vi "Update Class Properties.vi"(8 "error in (no error)":errorcluster, 11 "QControl Creation in":refnum<class "QControl Creation.lvclass">) -> (0 "error out":errorcluster, 3 "QControl Creation (dup)":refnum<class "QControl Creation.lvclass">)   [LabVIEW 2020, in "QControl Creation.lvclass"]
doc: "<b> </b> <b> </b>\n©2016 Q Software Innovations, LLC (QSI)\nwritten by Quentin Alldredge\nproduced in LabVIEW 2015\n\nsupport@qsoftwareinnovations.com\nwww.qsoftwareinnovations.com\n\nAll rights reserved.\n\nRedistribution and use in source and binary forms, with or without modification, are permitted provided that the following conditions are met:\n\n * Redistributions of source code must retain the above copyright notice, this list of conditions and the following disclaimer.\n * Redistributions in binary form must reproduce the above copyright notice, this list of conditions and the following disclaimer in the documentation and/or other materials provided with the distribution.\n * Neither the name of Q Software Innovations, LLC. nor the names of its contributors may be used to endorse or promote products derived from this software without specific prior written permission.\n\nTHIS SOFTWARE IS PROVIDED BY THE COPYRIGHT HOLDERS AND CONTRIBUTORS \"AS IS\" AND ANY EXPRESS OR IMPLIED WARRANTIES, INCLUDING, BUT NOT LIMITED TO, THE IMPLIED WARRANTIES OF MERCHANTABILITY AND FITNESS FOR A PARTICULAR PURPOSE ARE DISCLAIMED. IN NO EVENT SHALL THE COPYRIGHT OWNER OR CONTRIBUTORS BE LIABLE FOR ANY DIRECT, INDIRECT, INCIDENTAL, SPECIAL, EXEMPLARY, OR CONSEQUENTIAL DAMAGES (INCLUDING, BUT NOT LIMITED TO, PROCUREMENT OF SUBSTITUTE GOODS OR SERVICES; LOSS OF USE, DATA, OR PROFITS; OR BUSINESS INTERRUPTION) HOWEVER CAUSED AND ON ANY THEORY OF LIABILITY, WHETHER IN CONTRACT, STRICT LIABILITY, OR TORT (INCLUDING NEGLIGENCE OR OTHERWISE) ARISING IN ANY WAY OUT OF THE USE OF THIS SOFTWARE, EVEN IF ADVISED OF THE POSSIBILITY OF SUCH DAMAGE."
uses:
  QControl Creation.lvclass
  QControl Creation.lvclass/QControl Creation.ctl
  New QControl Info/New QControl Info.lvclass/New QControl Info.ctl
  New QControl Info/Read Localized Name.vi
  New QControl Info/Read Description.vi
  <vilib>/Utility/error.llb/Error Cluster From Error Code.vi
  <vilib>/ErrorRing/Error Ring.xnode
  New QControl Info/New QControl Info.lvclass
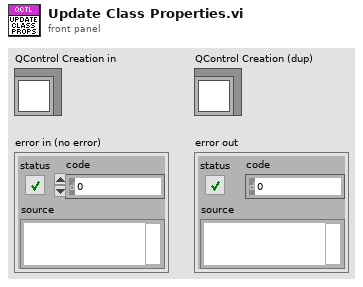
[diagram p1: front panel]
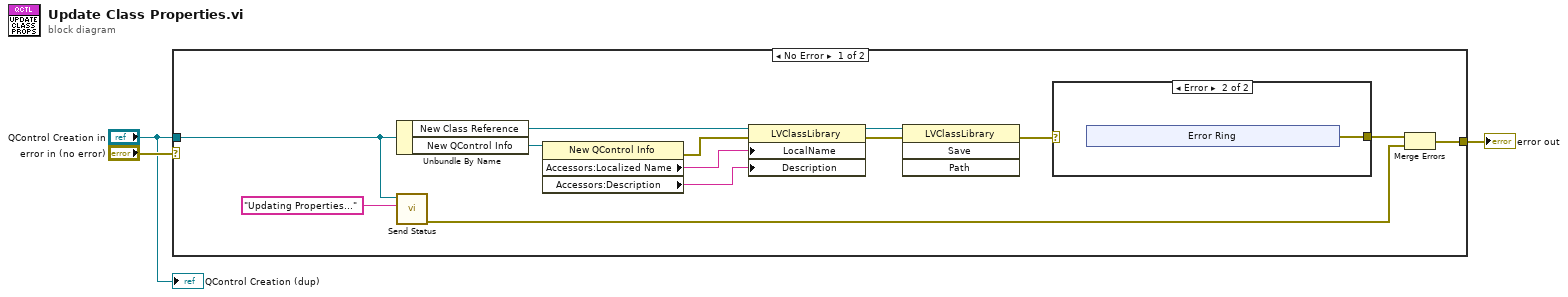
[diagram p0: block diagram]
diagram:
  n1 = case shown="No Error" "error in (no error)" {
    selector: "error in (no error)" -> [_ w24]
    tunnel: [w10 w24] -> w2
    tunnel: "QControl Creation in" -> [w11 _]
    frame No Error {
      n2 = Unbundle By Name(w11) -> ("New Class Reference"=w15:refnum<vi>, "New QControl Info"=w16:refnum<data-value>)
      n3 = call "Send Status.vi"("Status"="Updating Properties..." ("Value"), "QControl Creation in"=w11) -> ("error out (dup)"=w9:errorcluster)  [unwired: 8 in, 1 out]
      n4 = property class="New QControl Info"(reference=w16) -> (error out=w4:errorcluster, "Accessors:Localized Name"=w6:string, "Accessors:Description"=w5:string)  [unwired: 1 in, 1 out]
      n5 = property class="LVClassLibrary"(reference=w15, error in=w4, "LocalName"=w6, "Description"=w5) -> (reference out=w14:refnum<vi>, error out=w13:errorcluster)
      n6 = invoke class="LVClassLibrary" method="Save"(reference=w14, error in=w13) -> (error out=w7:errorcluster)  [unwired: 2 in, 3 out]
      n7 = case shown="Error" w7 {
        selector: w7 -> [w17 _]
        tunnel: [w17 w18] -> w8
        frame No Error {
        }
        frame Error {
          n8 = xnode "Error Ring"() -> ("error out"=w18:errorcluster)
        }
      }
      n9 = Merge Errors(w8, w9) -> (w10:errorcluster)
    }
    frame Error {
    }
  }
  "error out" <- w2
  "QControl Creation (dup)" <- "QControl Creation in"
